vi "scrollbar_min_max.vi"   [LabVIEW 2015, in "lv-graph.lvlib"]
uses:
  lv-graph.lvlib
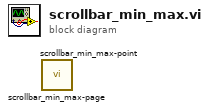
[diagram p0: block diagram]
diagram:
  n1 = call "scrollbar_min_max-page.vi"() -> ()  [unwired: 9 in, 3 out]
  n2 = call "scrollbar_min_max-point.vi"() -> ()  [unwired: 9 in, 3 out]
